vi "Actor Core.vi"(8 "error in":errorcluster, 11 "Basic Demo in":refnum<class "Basic Demo.lvclass">) -> (0 "error out":errorcluster, 3 "Actor out":refnum<class "Actor.lvclass">)   [LabVIEW 2017, in "2. Basic Panel Actors.lvlib" / "Basic Demo.lvclass"]
doc: "Allows the user to launch more panels of different types.\n----\nCopyright: MGI 2016\nAuthor: Derek Trepanier"
uses:
  Basic Demo.lvclass
  <vilib>/ActorFramework/Stop Msg/Stop Msg.lvclass
  Panel/Sample Panel.lvclass
  <vilib>/ActorFramework/Message Enqueuer/Message Enqueuer.lvclass
  Description Panel/Description Panel.lvclass
  panel-actors/Source/Panel Actor/Panel Actor.lvclass
  panel-manager/Source/MGI-Panel Manager.lvlib
  panel-manager/Source/Panel/Subpanel/Subpanel.vi
  panel-manager/Source/Panel/Subpanel/Subpanel.lvclass
  D:/software/LabView_PanelManager/panel-actors/Source/Panel Actor/Panel Actor.lvclass
  C:/Program Files (x86)/National Instruments/LabVIEW 2017/vi.lib/ActorFramework/Actor/Actor.lvclass
  panel-manager/Source/Panel/Window/Window.vi
  panel-manager/Source/Panel/Window/Window.lvclass
  panel-actors/Source/Panel Actor Messages/Show Panel Msg/Show Panel Msg.lvclass
  D:/software/LabView_PanelManager/panel-manager/Source/Panel/Panel.lvclass
  panel-manager/Source/Panel/Window/Dialog/Dialog.vi
  panel-manager/Source/Panel/Window/Dialog/Dialog.lvclass
  D:/software/LabView_PanelManager/panel-manager/Source/Panel/Window/Window.lvclass
  <vilib>/ActorFramework/Actor/Actor.lvclass
panel:
  in  "Show Window":bool
  in  "Show Dialog":bool
  in  "Running Sub-Panels":i32(listbox)
  in  "New Subpanel Item":bool
  # "Windows"
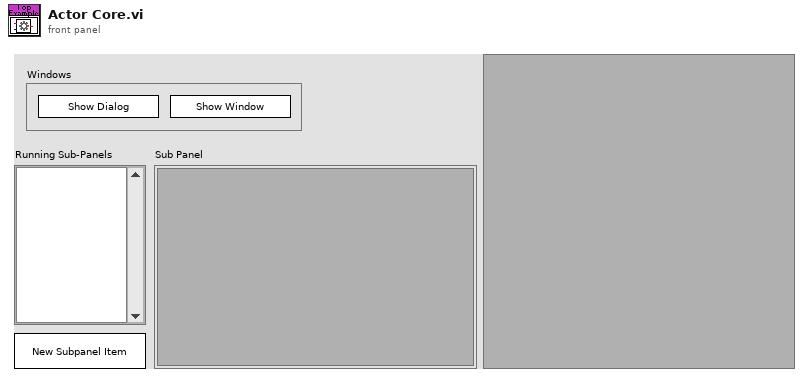
[diagram p1: front panel]
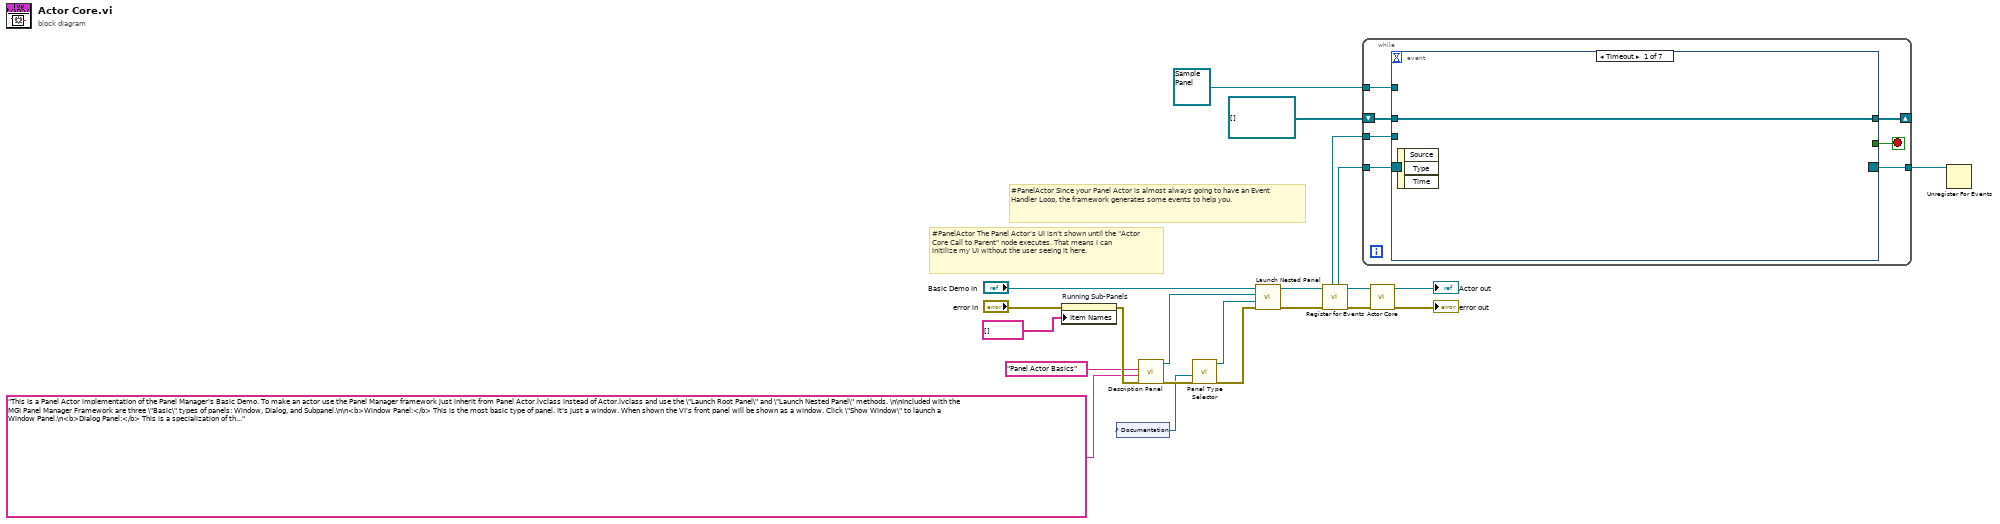
[diagram p0: block diagram]
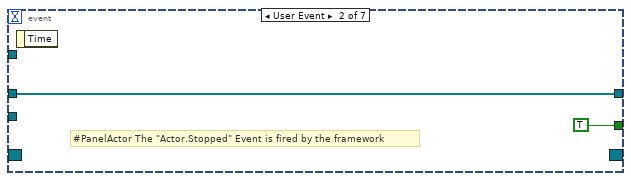
[diagram p2: hidden frame]
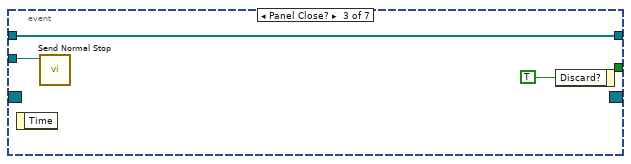
[diagram p3: hidden frame]
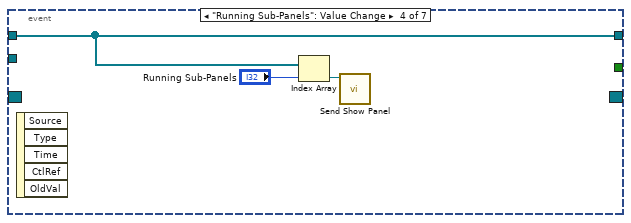
[diagram p4: hidden frame]
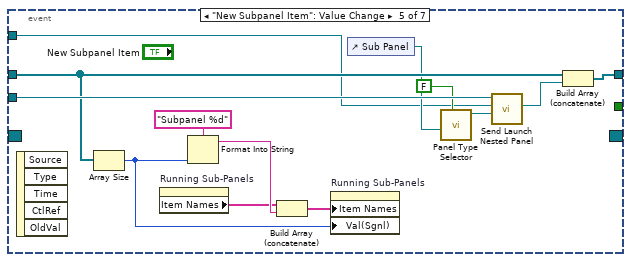
[diagram p5: hidden frame]
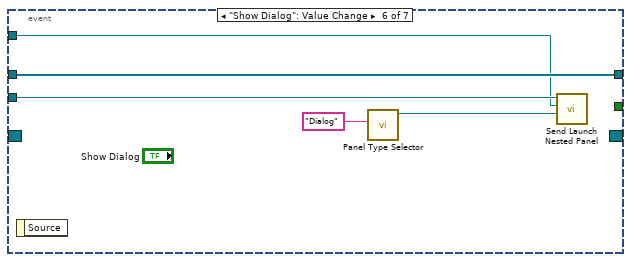
[diagram p6: hidden frame]
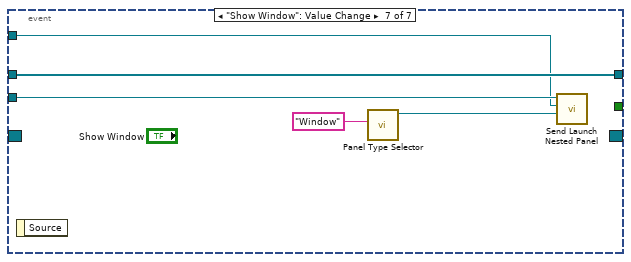
[diagram p7: hidden frame]
diagram:
  # "#PanelActor Since your Panel Actor is almost always going to have an Event Handler Loop, the framework generates some events to help you."
  # "#PanelActor The Panel Actor's UI isn't shown until the \"Actor Core Call to Parent\" node executes. That means I can initilize my UI without the user seeing it here."
  n1 = property on="Running Sub-Panels" class="LstBox (strict)"(error in="error in", "Item Names"=string[] []) -> (error out=w12:errorcluster)  [unwired: 1 in, 1 out]
  n2 = control-ref of="Documentation"() -> (w1:refnum<vi>)
  n3 = call "Description Panel.vi"("error in (no error)"=w12, "Description"="This is a Panel Actor implementation of the Panel Manager's Basic Demo. To make an actor use the Panel Manager framework just inherit from Panel Actor.lvclass instead of Actor.lvclass and use the \"Launch Root Panel\" and \"Launch Nested Panel\" methods. \n\nIncluded with the MGI Panel Manager Framework are three \"Basic\" types of panels: Window, Dialog, and Subpanel.\n\n<b>Window Panel:</b> This is the most basic type of panel. It's just a window. When shown the VI's front panel will be shown as a window. Click \"Show Window\" to launch a Window Panel.\n<b>Dialog Panel:</b> This is a specialization of the window panel. Again, the window will just be shown as a window, but the front panel will be set to modal. Click \"Show Dialog\" to launch a Dialog Panel.\n<b>Subpanel:</b> This panel type will insert the front panel into a subpanel of another VI. Click \"New Subpanel Item\" to launch a new Subpanel Panel. The list of running subpanel items is show in the \"Running Sub-Panels\" \n\nView the #PanelActor bookmark for more info.\n" ("Description Title"), "Description Title"="Panel Actor Basics") -> ("error out"=w11:errorcluster, "Description Panel out"=w8:refnum<class "Description Panel.lvclass">)  [unwired: 7 in]
  n4 = call-poly "Panel Type Selector.vi"("Error In"=w11, "Sub Panel"=w1) -> ("Error Out"=w10:errorcluster, "Subpanel Out"=w9:refnum<class "Subpanel.lvclass">)  [unwired: 8 in]
  n5 = call "Launch Nested Panel.vi"("error in (no error)"=w10, "Panel"=w9, "Nested Panel Actor"=w8, "Panel Actor in"="Basic Demo in") -> ("error out"=w13:errorcluster, "Panel Actor out"=w2:refnum<class "Basic Demo.lvclass">)  [unwired: 4 in, 2 out]
  n6 = call "Register for Events.vi"("Error In"=w13, "Panel Actor in"=w2) -> ("Error Out"=w21:errorcluster, "Panel Actor out"=w3:refnum<class "Basic Demo.lvclass">, "Pnl Actor"=w20:refnum<event-registration>, "Self Enqueuer"=w4:refnum<class "Message Enqueuer.lvclass">)  [unwired: 5 in, 1 out]
  n7 = while {
    tunnel: w20 -> [w29]
    tunnel: w4 -> [w28]
    shift-right: [w25] -> _
    shift-left: refnum<class "Message Enqueuer.lvclass">[] [] -> [w26]
    tunnel: refnum<class "Sample Panel.lvclass"> refnum ("Basic Panel Actors.lvlib:Panel.lvclass") -> [w24]
    tunnel: [w23] -> w5
    stop <- w27 stop-if-true
    n8 = event shown="[0] Timeout" {
      selector: w29 -> [_ _ _ _ _ _ _]
      dyn-events: [_ _ _ _ _ _ _] -> w23
      timeout: _ -> [_ _ _ _ _ _ _]
      tunnel: w28 -> [_ _ w34 _ w48 w55 w60]
      tunnel: [_ TRUE _ _ _ _ _] -> w27
      tunnel: w26 -> [w30 w31 w33 w38 w46 w56 w61]
      tunnel: [w30 w31 w33 w38 w51 w56 w61] -> w25
      tunnel: w24 -> [_ _ _ _ w39 w52 w57]
      event Timeout {
        n9 = event-data() -> ()  [unwired: 1 in, 3 out]
      }
      event User Event {
        # "#PanelActor The \"Actor.Stopped\" Event is fired by the framework"
        n10 = event-data() -> ()  [unwired: 1 in, 1 out]
      }
      event Panel Close? {
        n11 = event-data() -> ()  [unwired: 1 in, 1 out]
        n12 = call <vilib>:"Send Normal Stop.vi"("Message Enqueuer"=w34) -> ()  [unwired: 10 in, 1 out]
        n13 = event-data("Discard?"=TRUE) -> ()  [unwired: 1 in, 1 out]
      }
      event "Running Sub-Panels": Value Change {
        n14 = event-data() -> ()  [unwired: 1 in, 5 out]
        n15 = Index Array(array=w38, index="Running Sub-Panels") -> (element=w37:refnum<class "Message Enqueuer.lvclass">)
        n16 = call "Send Show Panel.vi"("Message Enqueuer in"=w37) -> ()  [unwired: 9 in, 2 out]
      }
      event "New Subpanel Item": Value Change {
        n17 = event-data() -> ()  [unwired: 1 in, 5 out]
        n18 = Array Size(array=w46) -> (size(s)=w42:i32)
        n19 = property on="Running Sub-Panels" class="LstBox (strict)"() -> ("Item Names"=w44:string[])  [unwired: 2 in, 2 out]
        n20 = Format Into String(format string="Subpanel %d", w42) -> (resulting string=w45:string)  [unwired: 2 in, 1 out]
        n21 = Build Array (concatenate)(w44, w45) -> (w43:string[])
        n22 = property on="Running Sub-Panels" class="LstBox (strict)"("Item Names"=w43, "Val(Sgnl)"=w42) -> ()  [unwired: 2 in, 2 out]
        n23 = control-ref of="Sub Panel"() -> (w40:refnum<vi>)
        n24 = call-poly "Panel Type Selector.vi"("Autoshow? (T)"=FALSE, "Sub Panel"=w40) -> ("Subpanel Out"=w49:refnum<class "Subpanel.lvclass">)  [unwired: 8 in, 1 out]
        n25 = call "Send Launch Nested Panel.vi"("Panel"=w49, "Nested Panel Actor"=w39, "Self Enqueuer in"=w48) -> ("Nested Actor's Enqueuer"=w50:refnum<class "Message Enqueuer.lvclass">)  [unwired: 6 in, 2 out]
        n26 = Build Array (concatenate)(w46, w50) -> (w51:refnum<class "Message Enqueuer.lvclass">[])
      }
      event "Show Dialog": Value Change {
        n27 = event-data() -> ()  [unwired: 1 in, 1 out]
        n28 = call-poly "Panel Type Selector.vi"("Default Title"="Dialog" ("Title")) -> ("Dialog out"=w54:refnum<class "Dialog.lvclass">)  [unwired: 9 in, 1 out]
        n29 = call "Send Launch Nested Panel.vi"("Panel"=w54, "Nested Panel Actor"=w52, "Self Enqueuer in"=w55) -> ()  [unwired: 6 in, 3 out]
      }
      event "Show Window": Value Change {
        n30 = event-data() -> ()  [unwired: 1 in, 1 out]
        n31 = call-poly "Panel Type Selector.vi"("Default Title"="Window" ("Title")) -> ("Window out"=w59:refnum<class "Window.lvclass">)  [unwired: 9 in, 1 out]
        n32 = call "Send Launch Nested Panel.vi"("Panel"=w59, "Nested Panel Actor"=w57, "Self Enqueuer in"=w60) -> ()  [unwired: 6 in, 3 out]
      }
    }
  }
  n33 = call-parent "Actor Core.vi"("error in"=w21, "Panel Actor in"=w3) -> ("error out"=→"error out":errorcluster, "Actor out"=→"Actor out":refnum<class "Actor.lvclass">)  [unwired: 8 in]
  n34 = Unregister For Events(event registration refnum=w5) -> ()  [unwired: 1 in, 1 out]
